vi "SaveVbreakTdm.vi"(0 "storage refnum (file)":refnum<k20>, 1 "Vbreak":dbl, 2 "Count":dbl, 3 "error in":errorcluster, 4 "Temp":dbl) -> (5 "storage refnum (file) 2":refnum<k20>, 6 "error out":errorcluster)   [LabVIEW 2014]
uses:
  <vilib>/Platform/storage/Storage.llb/usiSequenceRepresentation.ctl
  <vilib>/Platform/storage/Storage.llb/usiOverwriteOptions.ctl
  <vilib>/Platform/storage/lvStorage.llb/_createOrGetByNameExplicitChildObject.vi
  <vilib>/Platform/storage/Storage.llb/__savePropString.vi
  <vilib>/Platform/storage/lvStorage.llb/xStorage/xStorageSupp/ErrorOut.vi
  <vilib>/Platform/storage/lvStorage.llb/__saveFloat64Channel.vi
  <vilib>/Platform/storage/lvStorage.llb/xStorage/Write Data/Write Data.xnode
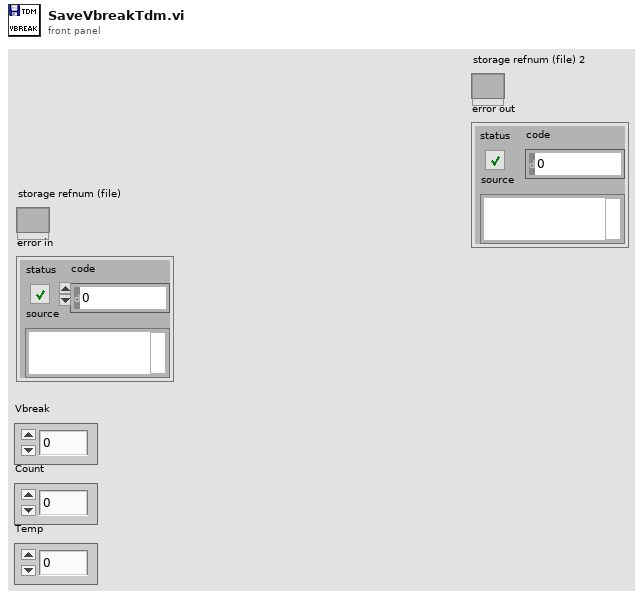
[diagram p1: front panel]
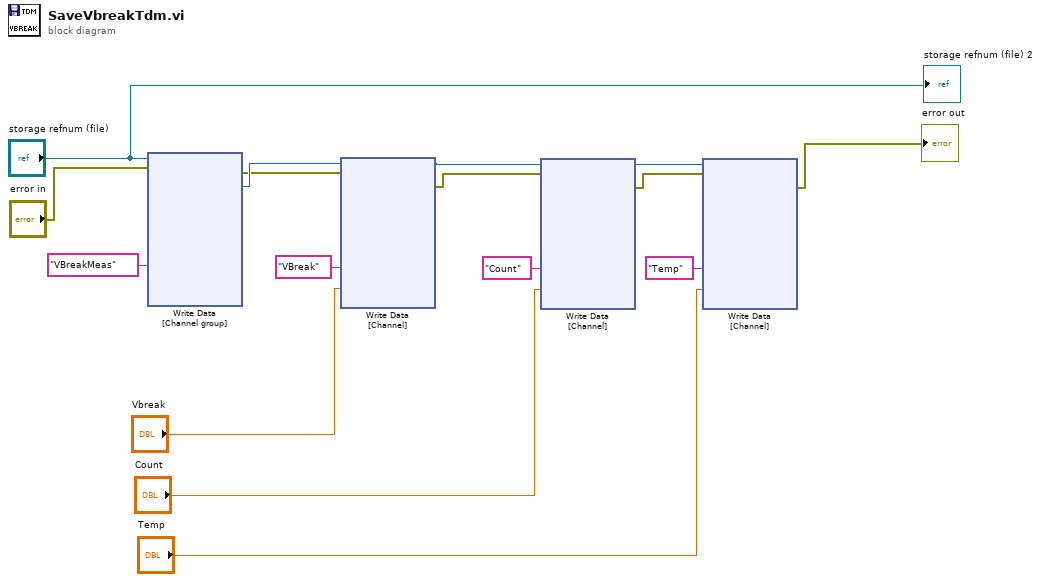
[diagram p0: block diagram]
diagram:
  n1 = xnode "Write Data\n[Channel group]"("Name"="VBreakMeas", "storage refnum (file)"="storage refnum (file)", "error in"="error in") -> ("error out"=w13:errorcluster, "storage refnum (channel group)"=w14:refnum<k20>)  [unwired: 1 in, 1 out]
  n2 = xnode "Write Data\n[Channel]"("Name"="VBreak", "Signal"="Vbreak", "storage refnum (channel group)"=w14, "error in"=w13) -> ("storage refnum (channel group) out"=w7:refnum<k20>, "error out"=w10:errorcluster)  [unwired: 2 in, 1 out]
  n3 = xnode "Write Data\n[Channel]"("Name"="Count", "Signal"="Count", "storage refnum (channel group)"=w7, "error in"=w10) -> ("storage refnum (channel group) out"=w6:refnum<k20>, "error out"=w5:errorcluster)  [unwired: 2 in, 1 out]
  n4 = xnode "Write Data\n[Channel]"("Name"="Temp", "Signal"="Temp", "storage refnum (channel group)"=w6, "error in"=w5) -> ("error out"=→"error out":errorcluster)  [unwired: 2 in, 2 out]
  "storage refnum (file) 2" <- "storage refnum (file)"
